vi "Init Edge Detector.vi"(6 "Unsee last word":bool=TRUE, 8 "error in (no error)":errorcluster, 11 "Spectrum Recorder too in":refnum<class "Spectrum Recorder too.lvclass">) -> (0 "error out":errorcluster, 3 "Spectrum Recorder too out":refnum<class "Spectrum Recorder too.lvclass">)   [LabVIEW 2024, in "Spectrum Recorder too.lvclass"]
uses:
  Spectrum Recorder too.lvclass
  Spectrum Recorder too.lvclass/Spectrum Recorder too.ctl
  Read RP transceiver.vi
  Write RP transceiver.vi
  NHMFL_Core/Libraries/Red Pitaya/RP Core/RP Transceiver/RP Transceiver.lvclass
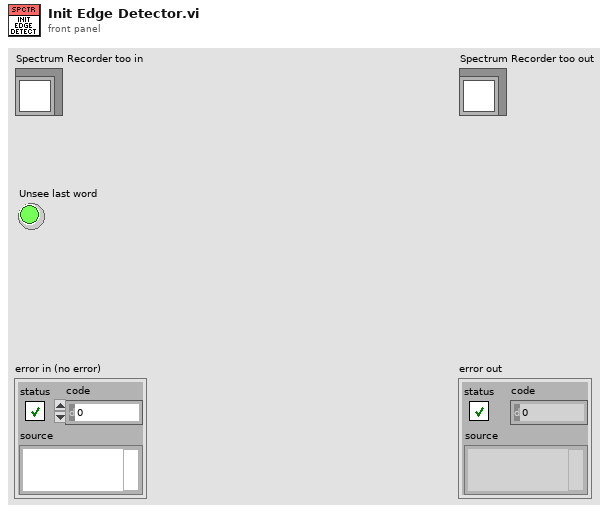
[diagram p1: front panel]
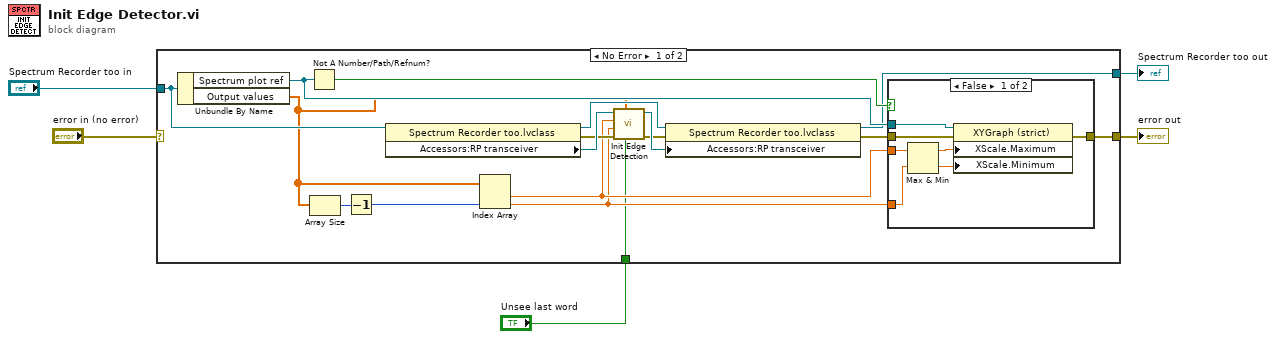
[diagram p0: block diagram]
diagram:
  n1 = case shown="No Error" "error in (no error)" {
    selector: "error in (no error)" -> [_ w32]
    tunnel: [w8 w32] -> w4
    tunnel: [w13 w31] -> w2
    tunnel: "Spectrum Recorder too in" -> [w14 w31]
    tunnel: "Unsee last word" -> [w7 _]
    frame No Error {
      n2 = Unbundle By Name(w14) -> ("Spectrum plot ref"=w19:refnum<vi>, "Output values"=w6:dbl[])
      n3 = Not A Number/Path/Refnum?(number/path/refnum=w19) -> (NaN/Path/Refnum?=w20:bool)
      n4 = Array Size(array=w6) -> (size(s)=w21:i32)
      n5 = Decrement(x=w21) -> (x-1=w22:i32)
      n6 = property class="Spectrum Recorder too.lvclass"(reference=w14) -> (reference out=w11:refnum<class "Spectrum Recorder too.lvclass">, error out=w16:errorcluster, "Accessors:RP transceiver"=w18:refnum<class "RP Transceiver.lvclass">)  [unwired: 1 in]
      n7 = Index Array(array=w6, index #2=w22) -> (element #1=w10:dbl, element #2=w9:dbl)  [unwired: 1 in]
      n8 = call-dynamic "Init Edge Detection.vi"("Unsee last word"=w7, "Output values"=w6, "error in (no error)"=w16, "Last output"=w9, "First output"=w10, "RP Transceiver in"=w18) -> ("error out"=w12:errorcluster, "RP Transceiver out"=w17:refnum<class "RP Transceiver.lvclass">)  [unwired: 4 in]
      n9 = property class="Spectrum Recorder too.lvclass"(reference=w11, error in=w12, "Accessors:RP transceiver"=w17) -> (reference out=w13:refnum<class "Spectrum Recorder too.lvclass">, error out=w15:errorcluster)
      n10 = case shown="False" w20 {
        tunnel: w19 -> [w29 _]
        tunnel: w15 -> [w28 w30]
        tunnel: w10 -> [w27 _]
        tunnel: w9 -> [w26 _]
        tunnel: [w23 w30] -> w8
        frame False {
          n11 = Max & Min(x=w27, y=w26) -> (max(x,y)=w25:dbl, min(x,y)=w24:dbl)
          n12 = property class="XYGraph (strict)"(reference=w29, error in=w28, "XScale.Maximum"=w25, "XScale.Minimum"=w24) -> (error out=w23:errorcluster)  [unwired: 1 out]
        }
        frame True {
        }
      }
    }
    frame Error {
    }
  }
  "error out" <- w4
  "Spectrum Recorder too out" <- w2
